vi "test Import Configuration File_VIV.vi"(8 "error in":errorcluster, 11 "TestCase in":refnum<class "Import.lvclass">) -> (0 "error out":errorcluster, 3 "TestCase out":refnum<class "Import.lvclass">)   [LabVIEW 2020, in "Import.lvclass"]
uses:
  Import.lvclass
  <vilib>/addons/_JKI Toolkits/VI Tester/TestCase.llb/TestCase.lvclass
  Import/ARINC 429 Import.lvlib
  niveristand-custom-device-testing-tools/VeriStandTestUtilities/VeriStandTestUtilities.lvlib
  C:/Program Files (x86)/National Instruments/LabVIEW 2020/vi.lib/addons/_JKI Toolkits/VI Tester/TestCase.llb/TestCase.lvclass
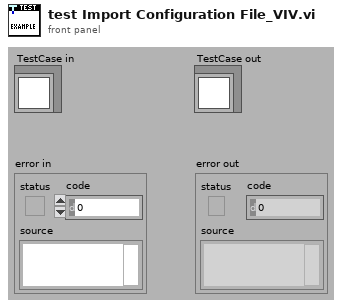
[diagram p1: front panel]
types:
  T1 = typedef "VS Channels Definition for All Labels on Hardware Channel.ctl" = cluster{"hardware channel":i32, "labels":T2[]}
  T2 = typedef "VS Channels Definition for Label.ctl" = cluster{"label (Dec)":i32, "parameters":T3[], "SDI value":u8, "SDI enabled":bool, "transfer type":T7}
  T3 = typedef "VS Channel Definition for Parameter.ctl" = cluster{"name":string, "direction":T4, "default value":dbl, "unit":string, "Parameter":T5}
  T4 = typedef "Direction.ctl" = enum16{"Rx", "Tx"}
  T5 = typedef "Parameter Definition.ctl" = cluster{"start index":i32, "size":i32, "encoding":T6, "signed":bool, "scale multiplier":dbl, "scale offset":dbl}
  T6 = typedef "Encoding and Decoding.lvlib/Encoding.ctl" = enum16{"BNR", "BCD", "Discrete"}
  T7 = typedef "Transfer Type.ctl" = enum16{"Scheduled", "Acyclic", "Block", "Strobe"}
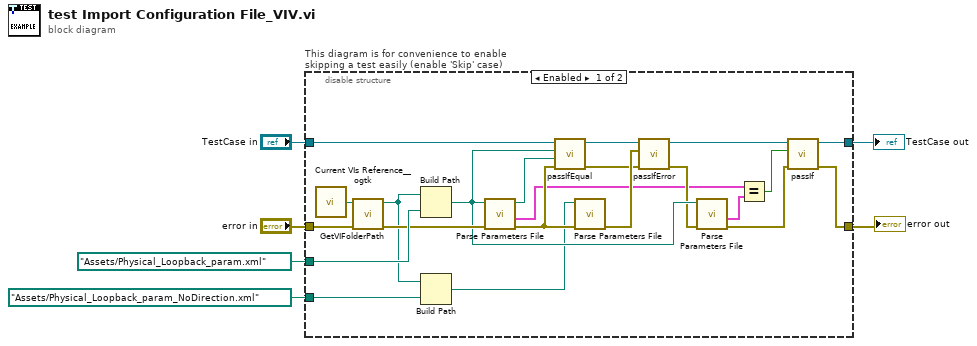
[diagram p0: block diagram]
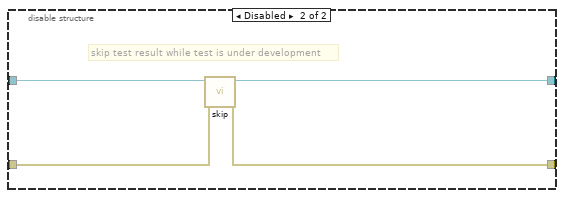
[diagram p2: hidden frame]
diagram:
  n1 = disable-structure "This diagram is for convenience to enable skipping a test easily (enable 'Skip' case)" shown="Enabled" {
    disable-tunnel: "TestCase in" -> [w28 w32]
    disable-tunnel: [w22 w30] -> w3
    disable-tunnel: [w23 w31] -> w5
    disable-tunnel: "error in" -> [w26 w29]
    disable-tunnel: path "Assets/Physical_Loopback_param.xml" ("Absolute or Relative Path") -> [w25 _]
    disable-tunnel: path "Assets/Physical_Loopback_param_NoDirection.xml" ("Absolute or Relative Path") -> [w18 _]
    frame Enabled {
      n2 = call <userlib>:"Current VIs Reference__ogtk.vi"() -> ("Current VI's reference"=w27:refnum<vi>)  [unwired: 5 in]
      n3 = call "GetVIFolderPath.vi"("error in (no error)"=w26, "VI Reference in"=w27) -> ("error out"=w24:errorcluster, "VI Folder Path out"=w19:path)  [unwired: 8 in]
      n4 = Build Path(base path=w19, name or relative path=w25) -> (appended path=w20:path)
      n5 = Build Path(base path=w19, name or relative path=w18) -> (appended path=w10:path)
      n6 = call "Parse Parameters File.vi"("error in"=w24, "path to XML document"=w20) -> ("error out"=w17:errorcluster, "ports"=w8:T1[], "path to XML document out"=w9:path)  [unwired: 7 in]
      n7 = call-dynamic "passIfEqual.vi"("error in (no error)"=w17, "y"=w9, "x"=w20, "TestCase in"=w28) -> ("error out"=w15:errorcluster, "TestCase out"=w14:refnum<class "Import.lvclass">)  [unwired: 6 in]
      n8 = call "Parse Parameters File.vi"("error in"=w17, "path to XML document"=w10) -> ("error out"=w16:errorcluster)  [unwired: 7 in, 2 out]
      n9 = call-dynamic "passIfError.vi"("error in (no error)"=w15, "error"=w16, "TestCase in"=w14) -> ("error out"=w12:errorcluster, "TestCase out"=w13:refnum<class "Import.lvclass">)  [unwired: 7 in]
      n10 = call "Parse Parameters File.vi"("error in"=w12, "path to XML document"=w20) -> ("error out"=w11:errorcluster, "ports"=w7:T1[])  [unwired: 7 in, 1 out]
      n11 = Equal?(x=w8, y=w7) -> (x = y?=w21:bool)
      n12 = call-dynamic "passIf.vi"("error in (no error)"=w11, "pass"=w21, "TestCase in"=w13) -> ("error out"=w23:errorcluster, "TestCase out"=w22:refnum<class "Import.lvclass">)  [unwired: 7 in]
    }
    frame Disabled {
      # "skip test result while test is under development"
      n13 = call <vilib>:"skip.vi"("error in (no error)"=w29, "TestCase in"=w32) -> ("error out"=w31:errorcluster, "TestCase out"=w30:refnum<class "Import.lvclass">)  [unwired: 8 in]
    }
  }
  "error out" <- w5
  "TestCase out" <- w3
